vi "Add Step Description.vi"(8 "error in (no error)":errorcluster, 10 "New Step Description":T1[](array[typedef]), 11 "Measurement Data in":refnum<class "Measurement Data.lvclass">) -> (0 "error out":errorcluster, 3 "Measurement Data out":refnum<class "Measurement Data.lvclass">)   [LabVIEW 2018, in "Measurement Data.lvlib" / "Measurement Data.lvclass"]
uses:
  Measurement Data.lvclass
  Controls/Measurement Description.ctl
  Plugins/String Database.lvlibp/String Database.lvclass
  Controls/Measurement Position.ctl
  Measurement Data.lvclass/Measurement Data.ctl
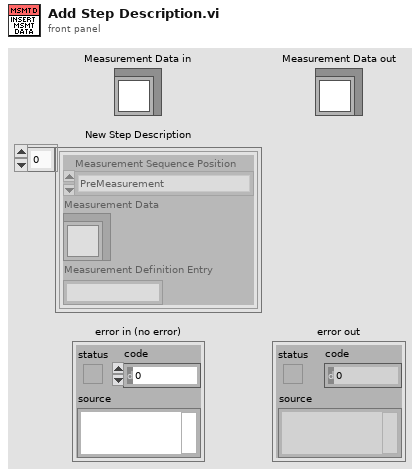
[diagram p1: front panel]
types:
  T1 = typedef "Measurement Data.lvlib/Measurement Data.lvclass/Measurement Description.ctl" = cluster{"Measurement Sequence Position":T2, "Measurement Data":refnum<class "String Database.lvclass">, "Measurement Definition Entry":string}
  T2 = typedef "Measurement Data.lvlib/Measurement Data.lvclass/Measurement Position.ctl" = enum16{"PreMeasurement", "MainMeasurement", "PostMeasurement"}
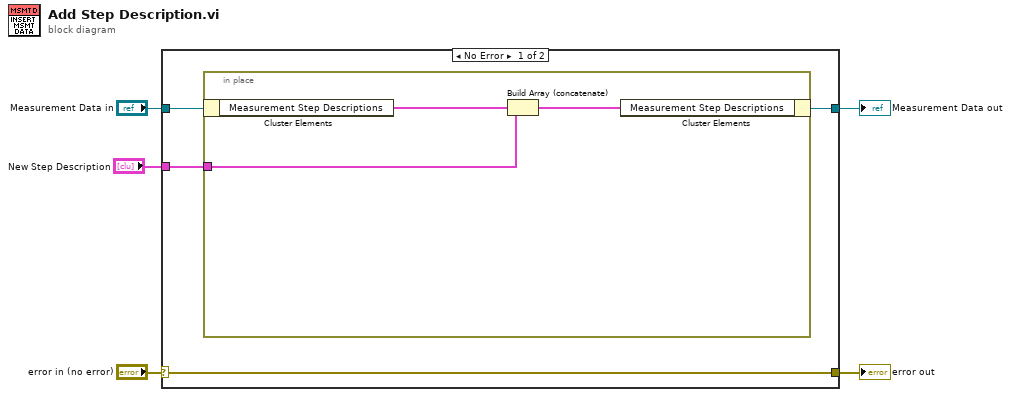
[diagram p0: block diagram]
diagram:
  n1 = case shown="No Error" "error in (no error)" {
    selector: "error in (no error)" -> [w9 w14]
    tunnel: [w9 w14] -> w4
    tunnel: [w7 w13] -> w2
    tunnel: "Measurement Data in" -> [w8 w13]
    tunnel: "New Step Description" -> [w6 _]
    frame No Error {
      n2 = in-place {
        in-place-border: w6 -> [w10]
        n3 = in-place-cluster #1(w8) -> ("Measurement Step Descriptions"=w12:T1[])
        n4 = Build Array (concatenate)(w12, w10) -> (w11:T1[])
        n5 = in-place-cluster #1("Measurement Step Descriptions"=w11) -> (w7:refnum<class "Measurement Data.lvclass">)
      }
    }
    frame Error {
    }
  }
  "error out" <- w4
  "Measurement Data out" <- w2
